vi "Laplace Random.vi"(6 "seed":i32=-1, 7 "reset":bool, 9 "b":dbl=1.0, 10 "a":dbl, 11 "samples":i32=128) -> (0 "error":i32, 3 "Laplace random numbers":dbl[](array[numeric]))   [LabVIEW 2010, in "NI_Gmath.lvlib"]
doc: "Generates random values from a variate X, where X describes the selected distribution type. You must manually select the polymorphic instance to use."
uses:
  NI_Gmath.lvlib
panel:
  # "Laplace Random"
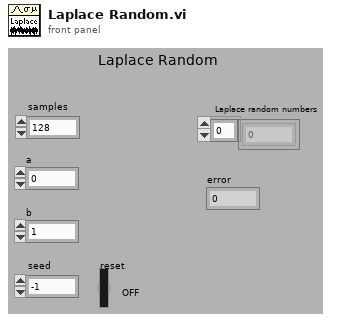
[diagram p1: front panel]
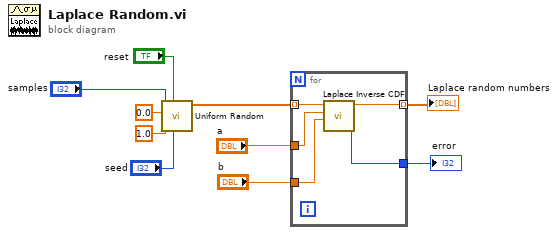
[diagram p0: block diagram]
diagram:
  n1 = call "Uniform Random.vi"("seed"="seed", "reset"="reset", "xmax"=1.0, "xmin"=0.0, "samples"="samples") -> ("uniform random data"=w3:dbl[])  [unwired: 5 in, 1 out]
  n2 = for {
    tunnel: w3 -> [w15] mode=indexing
    tunnel: "a" -> [w14]
    tunnel: "b" -> [w13]
    tunnel: [w12] -> w8 mode=indexing
    tunnel: [w11] -> w7
    n3 = call "Laplace Inverse CDF.vi"("b"=w13, "a"=w14, "cdf(x)"=w15) -> ("error"=w11:i32, "x"=w12:dbl)  [unwired: 7 in]
  }
  "error" <- w7
  "Laplace random numbers" <- w8
